vi "CreateAPI_VI.vi"(8 "error in (no error)":errorcluster, 10 "specific class reference":refnum<vi>, 11 "VI Refnum":refnum<vi>) -> (0 "error out":errorcluster)   [LabVIEW 2017]
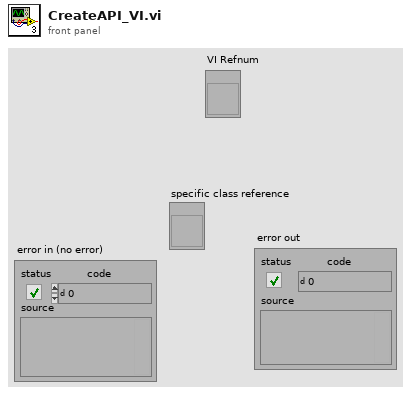
[diagram p1: front panel]
types:
  T1 = enum32{"invalid lock state", "Not Locked", "Locked (No Password)", "Password-protected"}
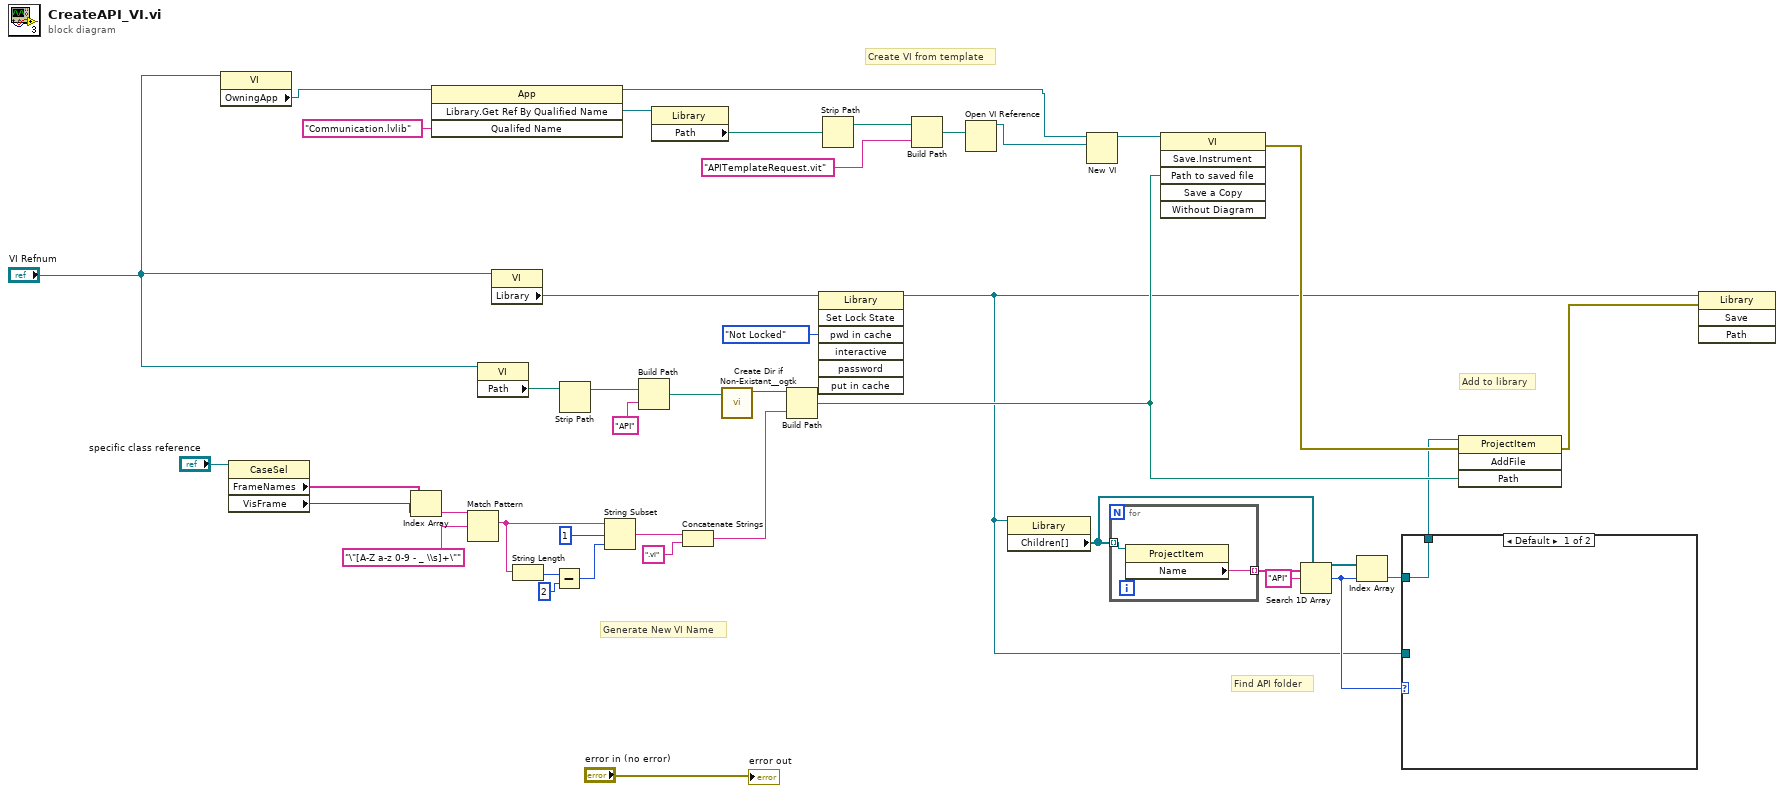
[diagram p0: block diagram]
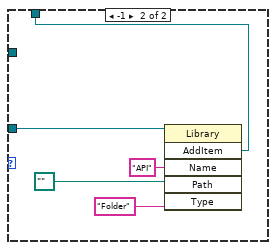
[diagram p2: hidden frame]
diagram:
  # "Add to library"
  # "Find API folder"
  # "Generate New VI Name"
  # "Create VI from template"
  n1 = property class="VI"(reference="VI Refnum") -> ("OwningApp"=w35:refnum<vi>)  [unwired: 1 in, 2 out]
  n2 = property class="CaseSel"(reference="specific class reference") -> ("FrameNames"=w28:string[], "VisFrame"=w27:u32)  [unwired: 1 in, 2 out]
  n3 = Index Array(array=w28, index=w27) -> (element=w20:string)
  n4 = invoke class="App" method="Library.Get Ref By Qualified Name"(reference=w35, "Qualifed Name"="Communication.lvlib" ("Qualified Name")) -> (reference out=w2:refnum<vi>, "Library.Get Ref By Qualified Name"=w41:refnum<vi>)  [unwired: 2 in, 2 out]
  n5 = Match Pattern(string=w20, regular expression="\"[A-Z a-z 0-9 - _ \\s]+\"") -> (match substring=w17:string)  [unwired: 1 in, 3 out]
  n6 = property class="VI"(reference="VI Refnum") -> ("Path"=w32:path)  [unwired: 1 in, 2 out]
  n7 = property class="VI"(reference="VI Refnum") -> ("Library"=w21:refnum<vi>)  [unwired: 1 in, 2 out]
  n8 = String Length(string=w17) -> (length=w16:i32)
  n9 = Subtract(x=w16, y=2) -> (x-y=w14:i32)
  n10 = Strip Path(path=w32) -> (stripped path=w31:path)  [unwired: 1 out]
  n11 = String Subset(string=w17, offset (0)=1, length (rest)=w14) -> (substring=w13:string)
  n12 = Build Path(base path=w31, name or relative path="API") -> (appended path=w30:path)
  n13 = property class="Library"(reference=w41) -> ("Path"=w40:path)  [unwired: 1 in, 2 out]
  n14 = Concatenate Strings(w13, ".vi" ("string")) -> (w25:string)
  n15 = call <userlib>:"Create Dir if Non-Existant__ogtk.vi"("Directory Path"=w30) -> ("dup Directory Path"=w29:path)  [unwired: 8 in, 2 out]
  n16 = Build Path(base path=w29, name or relative path=w25) -> (appended path=w12:path)
  n17 = invoke class="Library" method="Set Lock State"(reference=w21, "pwd in cache"=T1."Not Locked" ("lock state")) -> (reference out=w3:refnum<vi>)  [unwired: 5 in, 6 out]
  n18 = Strip Path(path=w40) -> (stripped path=w39:path)  [unwired: 1 out]
  n19 = Build Path(base path=w39, name or relative path="APITemplateRequest.vit") -> (appended path=w37:path)
  n20 = Open VI Reference(vi path=w37) -> (vi reference=w34:refnum<vi>)  [unwired: 5 in, 1 out]
  n21 = property class="Library"(reference=w3) -> ("Children[]"=w7:refnum<vi>[])  [unwired: 1 in, 2 out]
  n22 = New VI(10:w34, 11:w2) -> (3:w33:refnum<vi>)  [unwired: 5 in, 1 out]
  n23 = for {
    tunnel: w7 -> [w44] mode=indexing
    tunnel: [w43] -> w9 mode=indexing
    n24 = property class="ProjectItem"(reference=w44) -> ("Name"=w43:string)  [unwired: 1 in, 2 out]
  }
  n25 = invoke class="VI" method="Save.Instrument"(reference=w33, "Path to saved file"=w12) -> (error out=w11:errorcluster)  [unwired: 4 in, 5 out]
  n26 = Search 1D Array(1D array=w9, element="API") -> (index of element=w6:i32)  [unwired: 1 in]
  n27 = Index Array(array=w7, index=w6) -> (element=w5:refnum<vi>)
  n28 = case shown="Default" w6 {
    tunnel: w3 -> [_ w47]
    tunnel: w5 -> [w45 _]
    tunnel: [w45 w46] -> w4
    frame Default {
    }
    frame -1 {
      n29 = invoke class="Library" method="AddItem"(reference=w47, "Name"="API", "Path"=path "", "Type"="Folder" ("Name")) -> ("AddItem"=w46:refnum<vi>)  [unwired: 2 in, 5 out]
    }
  }
  n30 = invoke class="ProjectItem" method="AddFile"(reference=w4, error in=w11, "Path"=w12) -> (error out=w10:errorcluster)  [unwired: 1 in, 3 out]
  n31 = invoke class="Library" method="Save"(reference=w3, error in=w10) -> ()  [unwired: 2 in, 4 out]
  "error out" <- "error in (no error)"
